vi "Set IRead Image.vi"(10 "IRead Image":refnum<class "IRead Image.lvclass">, 11 "Worker in":refnum<class "Camera Worker.lvclass">) -> (3 "Worker out":refnum<class "Camera Worker.lvclass">)   [LabVIEW 2024, in "Camera Worker.lvlib" / "Camera Worker.lvclass"]
uses:
  Camera Worker.lvclass
  Interfaces/IRead Image/IRead Images/IRead Image.lvclass
  Camera Worker.lvclass/Camera Worker.ctl
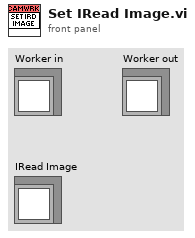
[diagram p1: front panel]
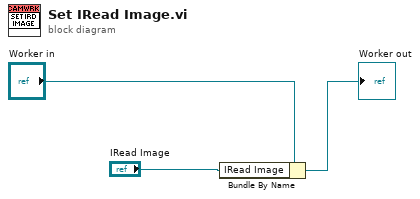
[diagram p0: block diagram]
diagram:
  n1 = Bundle By Name(cluster="Worker in", "IRead Image"="IRead Image") -> (→"Worker out":refnum<class "Camera Worker.lvclass">)
